vi "read_com.vi"(7 "wait sec":dbl=0.1 caption="等待时间(s)", 8 "error in":errorcluster caption="错误输入（无错误）", 9 "read bytes":u32 caption="读取字节数", 10 "write to buffer":string caption="写入缓冲区", 11 "VISA resource name in":refnum<visa-resource-name>="COM2") -> (0 "error out":errorcluster caption="错误输出", 1 "get bytes":u32 caption="返回字节数", 2 "read from buffer":string caption="读取缓冲区", 3 "VISA resource name out":refnum<visa-resource-name>="COM2")   [LabVIEW 2015]
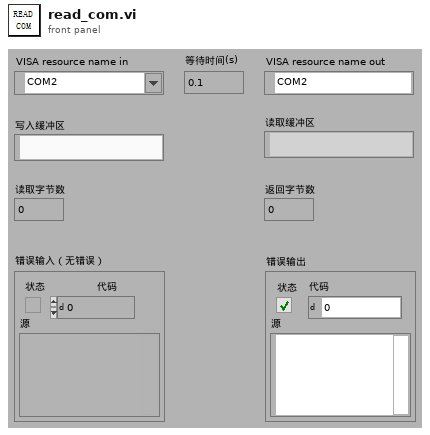
[diagram p1: front panel]
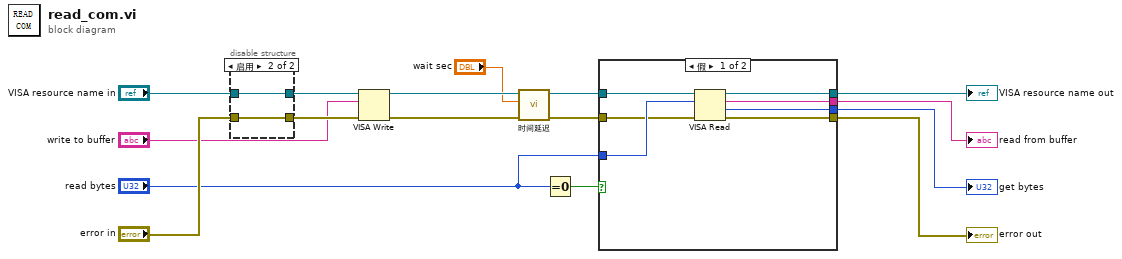
[diagram p0: block diagram]
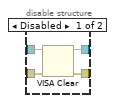
[diagram p2: hidden frame]
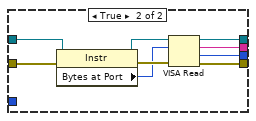
[diagram p3: hidden frame]
diagram:
  n1 = disable-structure shown="启用" {
    disable-tunnel: "VISA resource name in" -> [w19 w21]
    disable-tunnel: [w18 w21] -> w9
    disable-tunnel: "error in" -> [w17 w20]
    disable-tunnel: [w16 w20] -> w7
    frame Disabled {
      n2 = VISA Clear(VISA resource name=w19, error in (no error)=w17) -> (VISA resource name out=w18:refnum<visa-resource-name>, error out=w16:errorcluster)
    }
    frame Enabled {
    }
  }
  n3 = VISA Write(VISA resource name=w9, write buffer="write to buffer", error in (no error)=w7) -> (VISA resource name out=w14:refnum<visa-resource-name>, error out=w3:errorcluster)  [unwired: 1 out]
  n4 = call "时间延迟"("error in (no error)"=w3, "Delay Time (s)"="wait sec") -> ("error out"=w2:errorcluster)  [unwired: 9 in]
  n5 = Equal To 0?(x="read bytes") -> (x = 0?=w5:bool)
  n6 = case shown="假" w5 {
    tunnel: [w28 w37] -> w15
    tunnel: w14 -> [w27 w36]
    tunnel: [w26 w35] -> w13
    tunnel: [w25 w34] -> w12
    tunnel: [w24 w33] -> w10
    tunnel: w2 -> [w22 w31]
    tunnel: "read bytes" -> [w23 _]
    frame False {
      n7 = VISA Read(VISA resource name=w27, byte count=w23, error in (no error)=w22) -> (VISA resource name out=w25:refnum<visa-resource-name>, read buffer=w26:string, return count=w24:u32, error out=w28:errorcluster)
    }
    frame True {
      n8 = property class="Instr"(reference=w36, error in=w31) -> (reference out=w32:refnum<visa-resource-name>, error out=w30:errorcluster, "Bytes at Port"=w29:u32)
      n9 = VISA Read(VISA resource name=w32, byte count=w29, error in (no error)=w30) -> (VISA resource name out=w34:refnum<visa-resource-name>, read buffer=w35:string, return count=w33:u32, error out=w37:errorcluster)
    }
  }
  "error out" <- w15
  "read from buffer" <- w13
  "VISA resource name out" <- w12
  "get bytes" <- w10
